vi "Read Data DVR.vi"(8 "error in (no error)":errorcluster, 11 "cPAS Data DVR in":refnum<class "cPAS Data DVR.lvclass">) -> (0 "error out":errorcluster, 2 "Data DVR":refnum<data-value>, 3 "cPAS Data DVR out":refnum<class "cPAS Data DVR.lvclass">)   [LabVIEW 2015, in "cPAS Data DVR.lvclass"]
uses:
  cPAS Data DVR.lvclass
  Reusable/Data/Data.lvclass
  cPAS Data DVR.lvclass/cPAS Data DVR.ctl
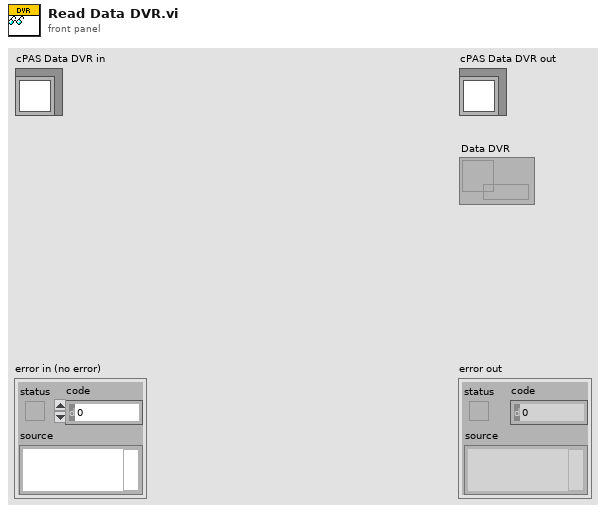
[diagram p1: front panel]
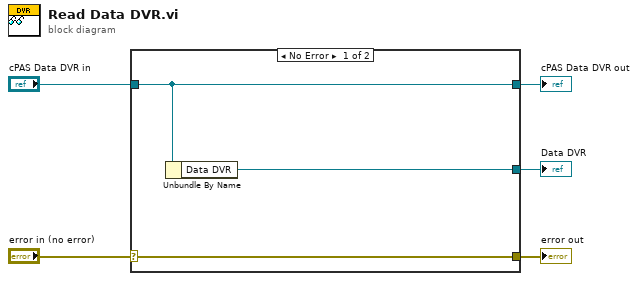
[diagram p0: block diagram]
diagram:
  n1 = case shown="No Error" "error in (no error)" {
    selector: "error in (no error)" -> [w8 w9]
    tunnel: [w8 w9] -> w4
    tunnel: [w7 w10] -> w2
    tunnel: "cPAS Data DVR in" -> [w7 w10]
    tunnel: [w6 _] -> w1
    frame No Error {
      n2 = Unbundle By Name(w7) -> ("Data DVR"=w6:refnum<data-value>)
    }
    frame Error {
    }
  }
  "error out" <- w4
  "cPAS Data DVR out" <- w2
  "Data DVR" <- w1
